vi "Launcher.vi"   [LabVIEW 2015]
uses:
  Actors/Calculator Actor/Calculator Actor Class/Calculator Actor.lvclass
  <vilib>/ActorFramework/Actor/Actor.lvclass
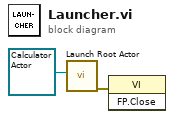
[diagram p0: block diagram]
diagram:
  n1 = call <vilib>:"Launch Root Actor.vi"("Actor"=refnum<class "Calculator Actor.lvclass"> refnum ("Calculator Actor.lvclass")) -> ("error out"=w1:errorcluster)  [unwired: 9 in, 1 out]
  n2 = invoke class="VI" method="FP.Close"(error in=w1) -> ()  [unwired: 2 in, 3 out]
